vi "Format Properties Table.vi"(8 "File Properties":string[][](array[string]), 9 "Group Properties":string[][](array[string]), 10 "Channel Properties":string[][](array[string]), 11 "Properties Table In":refnum<vi>) -> (2 "Properties Out":string[][](array[string]), 3 "Properties Table Out":refnum<vi>)   [LabVIEW 2017, in "XTree.xctl"]
doc: "Adds bolded headings to properties, shades sets of properties, and resets the scroll position of the properties table."
uses:
  <vilib>/addons/_NIFileIO/XTree/XTree.xctl
  <vilib>/Utility/miscctls.llb/LVRowAndColumnUnsignedTypeDef.ctl
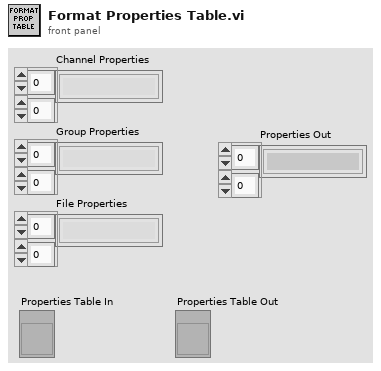
[diagram p1: front panel]
types:
  T1 = typedef "LVRowAndColumnTypeDef.ctl" = cluster{"Row":i32, "Column":i32}
  T2 = typedef "LVRowAndColumnUnsignedTypeDef.ctl" = cluster{"Row":u32, "Column":u32}
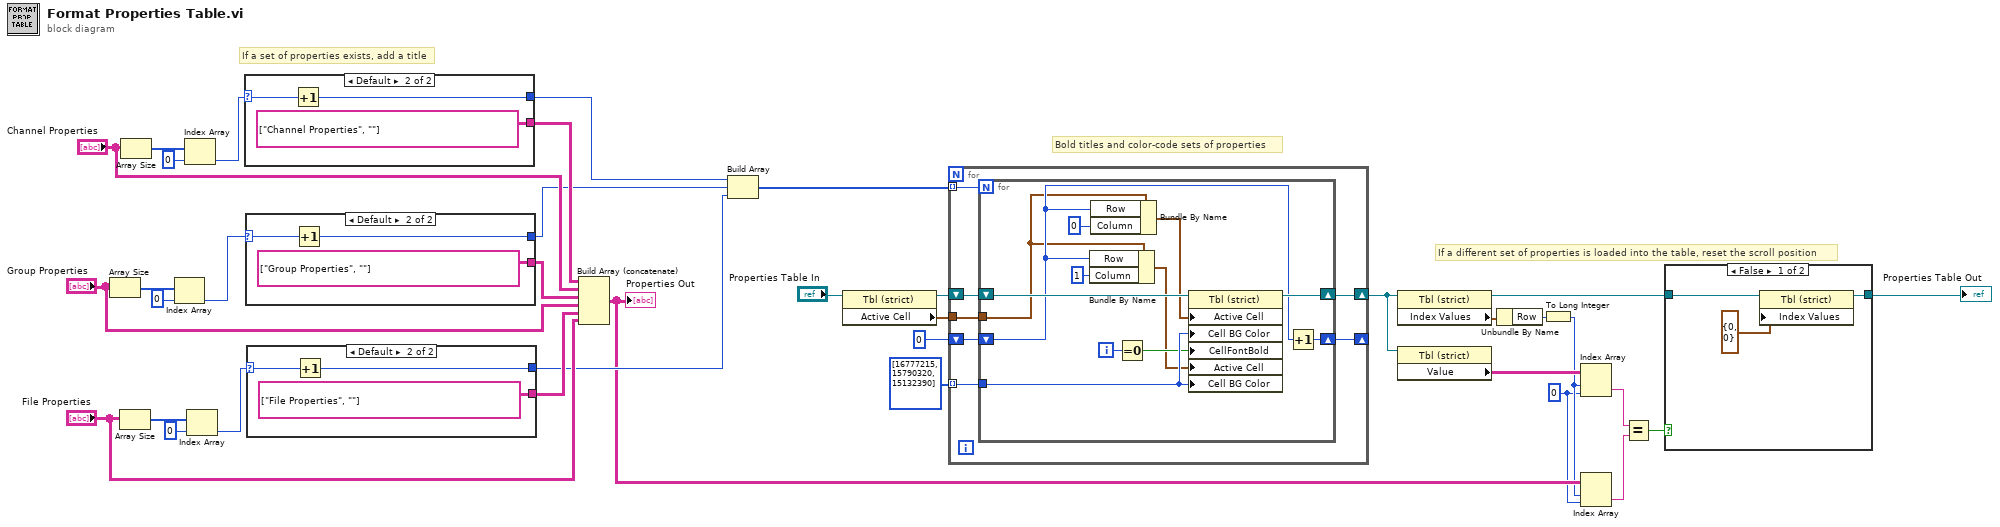
[diagram p0: block diagram]
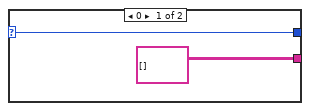
[diagram p3: hidden frame]
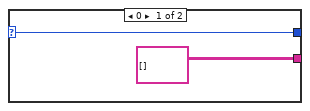
[diagram p4: hidden frame]
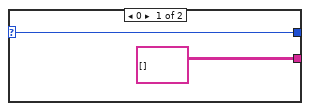
[diagram p5: hidden frame]
diagram:
  w6 = 0 ("disabled index (col)")
  # "If a different set of properties is loaded into the table, reset the scroll position"
  # "Bold titles and color-code sets of properties"
  # "If a set of properties exists, add a title"
  n1 = Array Size(array="Group Properties") -> (size(s)=w29:i32[])
  n2 = Array Size(array="File Properties") -> (size(s)=w24:i32[])
  n3 = Array Size(array="Channel Properties") -> (size(s)=w36:i32[])
  n4 = Index Array(array=w29, index=0) -> (element=w27:i32)
  n5 = Index Array(array=w36, index=0) -> (element=w32:i32)
  n6 = Index Array(array=w24, index=0) -> (element=w22:i32)
  n7 = case shown="Default" w32 {
    selector: w32 -> [w37 w40]
    tunnel: [string[][] [] ("t") string[][] [["Channel Properties", ""]]] -> w31
    tunnel: [w37 w39] -> w30
    frame 0 {
    }
    frame Default {
      n8 = Increment(x=w40) -> (x+1=w39:i32)
    }
  }
  n9 = case shown="Default" w27 {
    selector: w27 -> [w42 w45]
    tunnel: [string[][] [] ("t") string[][] [["Group Properties", ""]]] -> w25
    tunnel: [w42 w44] -> w21
    frame 0 {
    }
    frame Default {
      n10 = Increment(x=w45) -> (x+1=w44:i32)
    }
  }
  n11 = case shown="Default" w22 {
    selector: w22 -> [w47 w50]
    tunnel: [string[][] [] ("t") string[][] [["File Properties", ""]]] -> w20
    tunnel: [w47 w49] -> w13
    frame 0 {
    }
    frame Default {
      n12 = Increment(x=w50) -> (x+1=w49:i32)
    }
  }
  n13 = Build Array (concatenate)(w31, "Channel Properties", w25, "Group Properties", w20, "File Properties") -> (w8:string[][])
  "Properties Out" <- w8
  n14 = Build Array(w30, w21, w13) -> (w33:i32[])
  n15 = property class="Tbl (strict)"(reference="Properties Table In") -> (reference out=w14:refnum<vi>, "Active Cell"=w15:T1)  [unwired: 1 in, 1 out]
  n16 = for {
    tunnel: w33 -> [w58] mode=indexing
    shift-right: [w56] -> _
    shift-left: 0 -> [w57]
    tunnel: u32[] [16777215, 15790320, 15132390] -> [w55] mode=indexing
    shift-right: [w54] -> w12
    shift-left: w14 -> [w52]
    tunnel: w15 -> [w53]
    n17 = for {
      N: w58 -> [_]
      shift-right: [w70] -> w56
      shift-left: w57 -> [w60]
      tunnel: w55 -> [w68]
      shift-right: [w69] -> w54
      shift-left: w52 -> [w65]
      tunnel: w53 -> [w59]
      i -> [w67]
      n18 = Bundle By Name(cluster=w59, "Row"=w60, "Column"=1) -> (w62:T1)
      n19 = Bundle By Name(cluster=w59, "Row"=w60, "Column"=0) -> (w63:T1)
      n20 = Equal To 0?(x=w67) -> (x = 0?=w66:bool)
      n21 = property class="Tbl (strict)"(reference=w65, "Active Cell"=w63, "Cell BG Color"=w68, "CellFontBold"=w66, "Active Cell"=w62, "Cell BG Color"=w68) -> (reference out=w69:refnum<vi>)  [unwired: 1 in, 1 out]
      n22 = Increment(x=w60) -> (x+1=w70:i32)
    }
  }
  n23 = property class="Tbl (strict)"(reference=w12) -> (reference out=w2:refnum<vi>, "Index Values"=w10:T2)  [unwired: 1 in, 1 out]
  n24 = property class="Tbl (strict)"(reference=w12) -> ("Value"=w11:string[][])  [unwired: 1 in, 2 out]
  n25 = Unbundle By Name(w10) -> ("Row"=w9:u32)
  n26 = To Long Integer(number=w9) -> (32bit integer=w7:i32)
  n27 = Index Array(array=w11, index (row)=w7, index (col)=w6) -> (element=w5:string)
  n28 = Index Array(array=w8, index (row)=w7, index (col)=w6) -> (element=w4:string)
  n29 = Equal?(x=w5, y=w4) -> (x = y?=w3:bool)
  n30 = case shown="False" w3 {
    tunnel: w2 -> [w73 w74]
    tunnel: [w72 w74] -> w1
    frame False {
      n31 = property class="Tbl (strict)"(reference=w73, "Index Values"=T2 {"Row"=0, "Column"=0}) -> (reference out=w72:refnum<vi>)  [unwired: 1 in, 1 out]
    }
    frame True {
    }
  }
  "Properties Table Out" <- w1
